vi "Scope_5782_AM_PID.vi"() -> ()   [LabVIEW 2013]
uses:
  <vilib>/userdefined/High Color/nirio_resource_hc.ctl
  FPGA/DataMode.ctl
  <vilib>/Analysis/4window.llb/windowTd.ctl
  Host/Scope/controls/power_spectrum_unit.ctl
  Host/Scope5782/Scope/controls/5782_trigger_type.ctl
  Host/Scope/controls/Data_calc_mode.ctl
  Host/Scope/controls/Data_display_mode.ctl
  Host/Scope/controls/Graph_references.ctl
  Host/Scope/controls/graph_controls.ctl
  Host/Scope/controls/Channel_select.ctl
  Host/Scope5782/Config/FPGAref_5782.ctl
  Host/Communication/response.ctl
  Host/Communication/driver_status.ctl
  Host/Communication/Driver/RemoteConnection/RemoteReferences.ctl
  Host/Communication/Driver/TcpServerDriver/TcpServerDriver.lvclass
  Host/Scope/controls/ScopeMode.ctl
  FPGA/fpga_settings.ctl
  Host/Communication/global_stop.vi
  <vilib>/FPGAPlugInAG/PXIe-7975R/niLvFpga_Open_PXIe-7975R.vi
  <vilib>/rvi/interface/common/dynamic/niFpgaDynamicAddResources.vi
  <vilib>/rvi/interface/common/niFpgaWaitOnOcc.vi
  <vilib>/Utility/error.llb/Error Cluster From Error Code.vi
  <vilib>/rvi/errors/niLvFpgaAdjustHostInterfaceError.vi
  <vilib>/FPGAPlugInAG/Dynamic/niLvFpga_Close_Dynamic.vi
  <vilib>/rvi/interface/nirviOpenFPGA/nirviOpenFPGA.xnode
  FPGA Bitfiles/FPGAmain5782_AM_PID_Tz+TpvSTxoU.lvbitx
  <vilib>/rvi/interface/nirviReadWriteControl/nirviReadWriteControl.xnode
  <vilib>/rvi/FXPMathLib/FxpInterpret/XNode/nifxpmath_Interpret.xnode
  <vilib>/rvi/interface/nirviMethod/nirviMethod.xnode
  <vilib>/rvi/interface/nirviCloseFPGA/nirviCloseFPGA.xnode
  Host/Utilities/Ticker/Ticker.lvclass
  NiFpgaLv.dll
  <vilib>/rvi/interface/Simulation/niFpgaSimulationCallBeginRW.vi
  Host/Communication/Driver/RemoteConnection/RemoteConnection.lvclass
  <vilib>/FPGAPlugInAG/Dynamic/niLvFpga_WriteFifo_Dynamic.vi
  <vilib>/rvi/errors/niLvFpgaMergeErrorWithErrorCode.vi
  <vilib>/Analysis/NI_AALPro.lvlib
panel:
  in  "Ch1 deltaF":bool
  in  "Ch0 deltaF":bool
  in  "Kp":fxp<+/-,32,4>
  in  "Kd/T":fxp<+/-,32,4>
  in  "Ki*T":fxp<+/-,32,4>
  in  "Feedback":bool
  in  "#bins":i32=1 min=1 max=16
  in  "ch1 DC offset":dbl caption="DC offset\nChannel 1"
  in  "ch0 DC offset":dbl caption="DC offset\nChannel 0"
  in  "Output delay delta":dbl(slide) scale=0.0..6.0
  in  "Output delay":dbl(slide) scale=0.0..6.0
  in  "Chart length":i32=200000
  in  "Trigmode":enum32{"Triggered", "Continuous"}(radio)
  in  "Refence for phase":T1
  in  "Graph_refs":T2
  out "Lower chart":dbl[][](graph)
  out "Upper chart":dbl[][](graph)
  out "Lower graph":i16[][](graph)
  in  "Buffer":T4
  in  "Display":T5
  in  "Output mixer fequency [MHz]":dbl
  in  "Trigger":T6
  in  "Ch1 Q":bool
  in  "Ch1 I":bool
  in  "Ch0 Q":bool
  in  "Ch0 I":bool
  in  "Ch1":bool
  in  "Ch0":bool
  out "stop 2":bool
  in  "Zoom freq X":bool
  in  "Zoom freq Y":bool
  in  "Zoom time Y":bool
  in  "Zoom time X":bool
  in  "Unit":T7
  in  "Window":T8=1 items=["Rectangle"=0, "Hanning"=1, "Hamming"=2, "Blackman-Harris"=3, "Exact Blackman"=4, "Blackman"=5, "Flat Top"=6, "4 Term B-Harris "=7, "7 Term B-Harris"=8, "Low Sidelobe"=9, "Blackman Nuttall"=11, "Triangle"=30, "Bartlett-Hanning"=31, "Bohman"=32, "Parzen"=33, "Welch"=34, "Kaiser"=60, "Dolph-Chebyshev"=61, "Gaussian"=62]
  in  "Samples per 5782 record":i32
  in  "Phase offset (deg)":dbl
  in  "Fequency [MHz]":dbl format="%#_8g"
  in  "Mode":T9
  in  "Mixer freq [MHz]":dbl
  out "freqdata":cluster{"f0":dbl, "df":dbl, "magnitude":dbl[]}[](graph)
  out "Upper graph":i16[][](graph)
  in  "Rumode":bool
  in  "Singleshot":bool
  out "error IO":errorcluster
  in  "stop":bool
  in  "resource name":T10="RIO0"
  out "Clocking Option Configured?":bool
  out "Configured?":bool
  # "FPGA setup"
  # "V"
  # "V"
  # "Output delay"
  # "ns"
  # "Auto Zoom"
  # "Output delay delta"
  # "ps"
  # "5782"
  # "Simulated data"
  # "FFT"
  # "Auto Zoom"
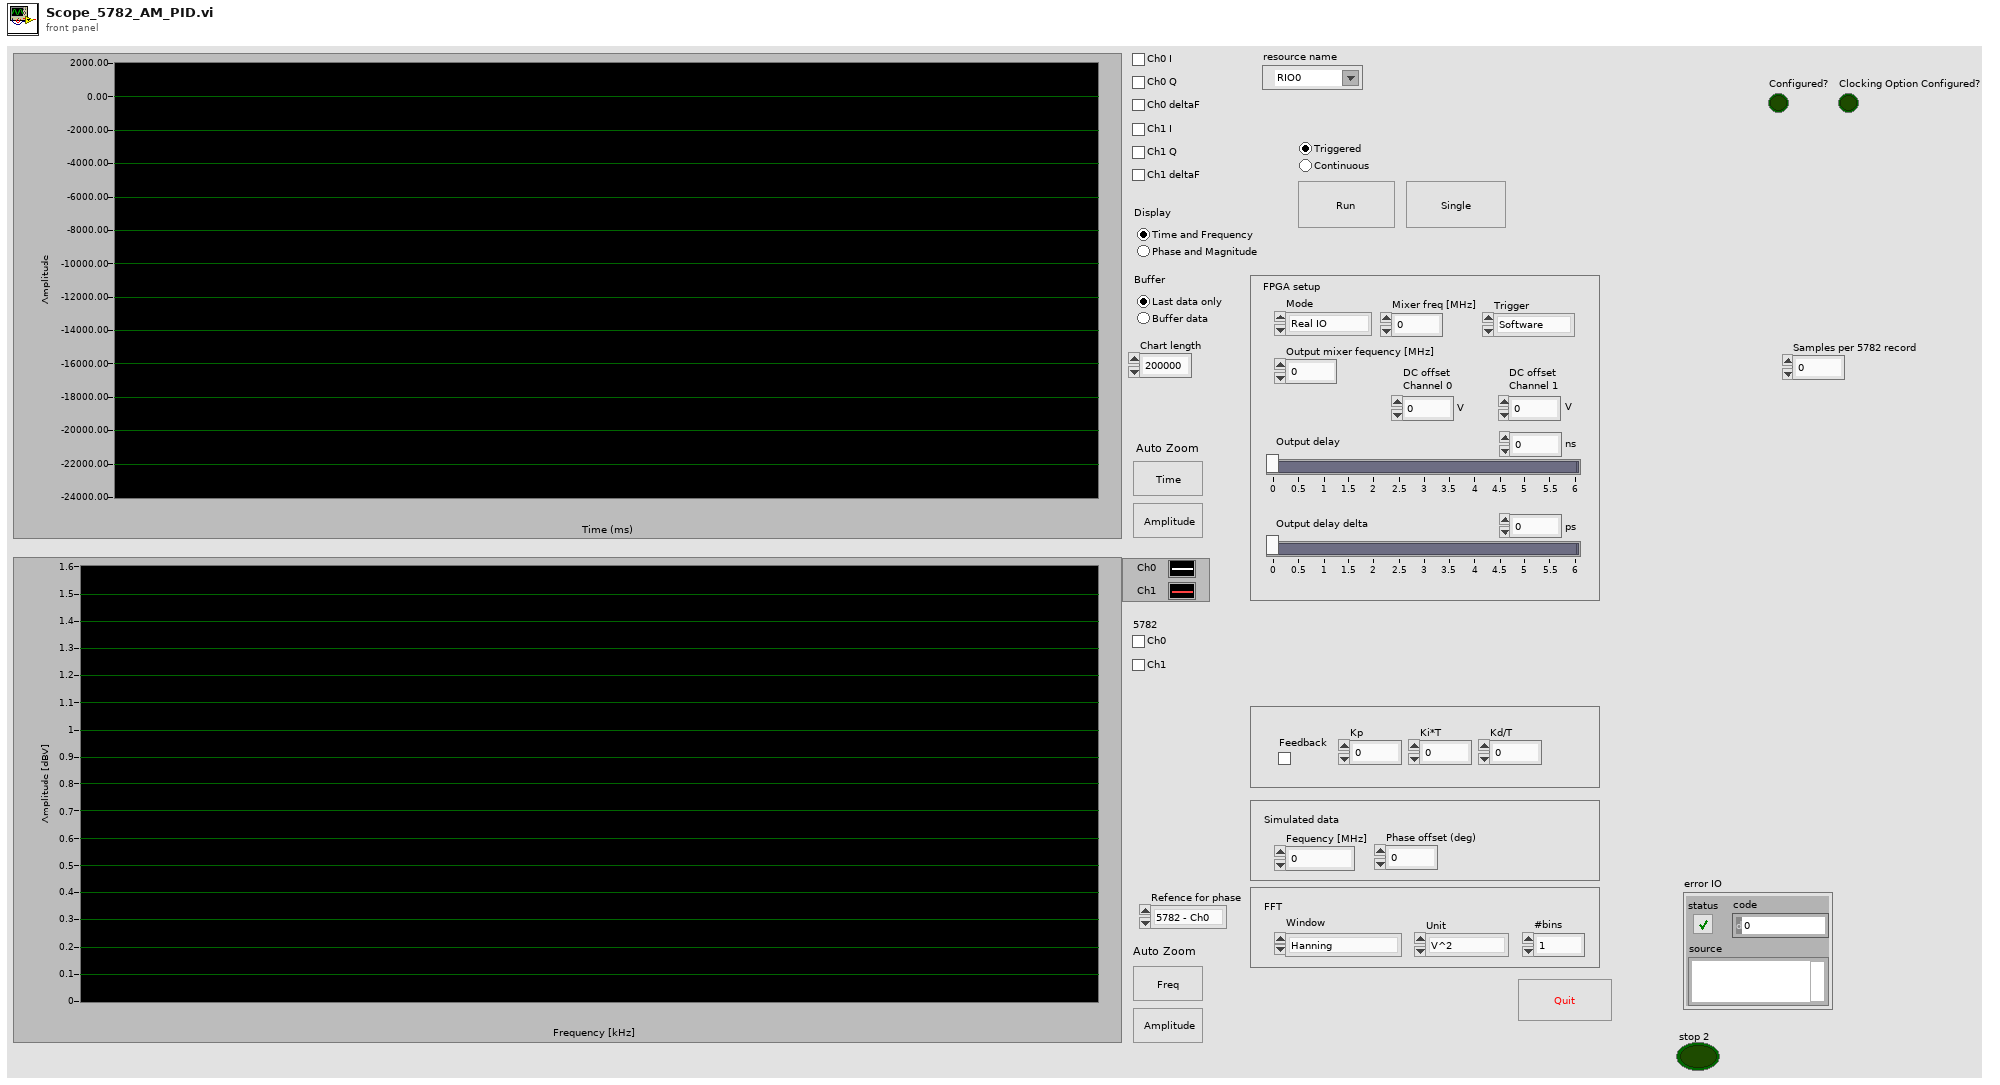
[diagram p1: front panel]
types:
  T1 = typedef "Channel_select.ctl" = enum16{"5782 - Ch0", "5782 - Ch1"}
  T2 = typedef "Graph_references.ctl" = cluster{"upper":T3, "lower":T3, "Freq graph":refnum<vi>}
  T3 = typedef "graph_controls.ctl" = cluster{"Graph":refnum<vi>, "Time btn":refnum<vi>, "Amplitude btn":refnum<vi>, "Chart":refnum<vi>}
  T4 = typedef "Data_display_mode.ctl" = enum32{"Last data only", "Buffer data"}
  T5 = typedef "Data_calc_mode.ctl" = enum32{"Time and Frequency", "Phase and Magnitude"}
  T6 = typedef "5782_trigger_type.ctl" = enum16{"Software", "Trigger input"}
  T7 = typedef "power_spectrum_unit.ctl" = enum16{"V^2", "V", "dBV"}
  T8 = typedef "NI_AALPro.lvlib/windowTd.ctl" = u32
  T9 = typedef "DataMode.ctl" = enum16{"Real IO", "Simulated"}
  T10 = typedef "nirio_resource_hc.ctl" = tag
  T11 = typedef "RemoteConnection.lvclass/RemoteReferences.ctl" = cluster{"a":refnum<vi>, "b":refnum<vi>, "fm":refnum<vi>, "Output delay":refnum<vi>, "Output delay delta":refnum<vi>}
  T12 = typedef "response.ctl" = cluster{"driver status":T13, "Sender":string, "Type":i32, "Variant":variant}
  T13 = typedef "driver_status.ctl" = enum16{"Normal", "Startup", "Connection lost", "Reconnected", "Timeout", "Idle", "Busy"}
  T14 = typedef "FPGAref_5782.ctl" = refnum<k20>
  T15 = enum8{"Internal Clock PLL Off", "Internal Clock PLL On (REF IN)", "External Clock (CLK_IN)", "Internal Clock PLL On (IoModSyncClk)"}
  T16 = typedef "message_queue.ctl" = refnum<queue>
  T17 = typedef "scope_params_5782.ctl" = cluster{"scope mode":T18, "ticker":refnum<class "Ticker.lvclass">, "samples per record":i32, "FPGA ref":T14, "data mode":T9, "5782 Trigger":T6, "Chart length":i32, "RemoteConnection":refnum<class "RemoteConnection.lvclass">, "last phase":dbl[]}
  T18 = typedef "ScopeMode.ctl" = enum16{"Stopped", "Single", "Running", "Continuous"}
  T19 = typedef "fpga_settings.ctl" = enum16{"Feedback Enable", "New FIR coeffs", "FIR shift", "Enable filter", "Set Downsample", "Downsample", "CIC Gain", "Record length", "Trigger samples", "Quiet time", "a_am", "b_am", "Use fixed delay", "fixed sin_fi", "fixed cos_fi", "Ki*Tau", "Kp", "Kd_Tau", "Fi_start", "Fi_delta", "DC_offs 0", "DC_offs 1", "Ki*Tau am", "Kp am", "Kd_Tau am"}
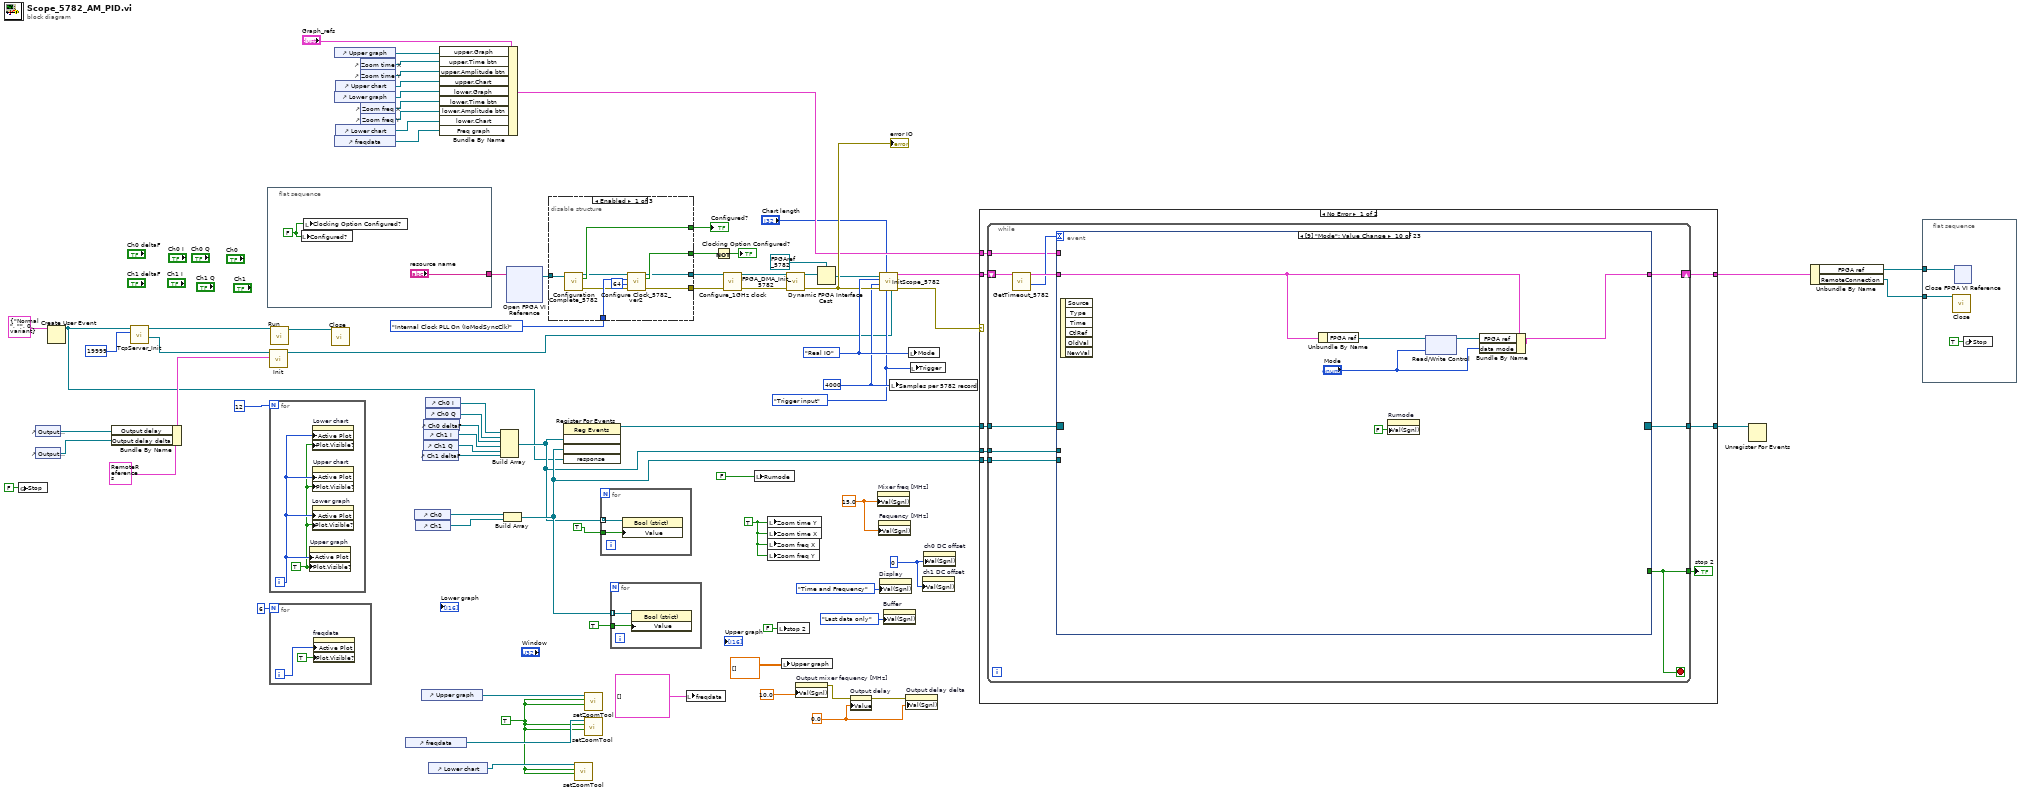
[diagram p0: block diagram]
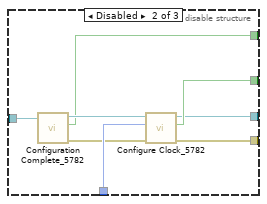
[diagram p2: hidden frame]
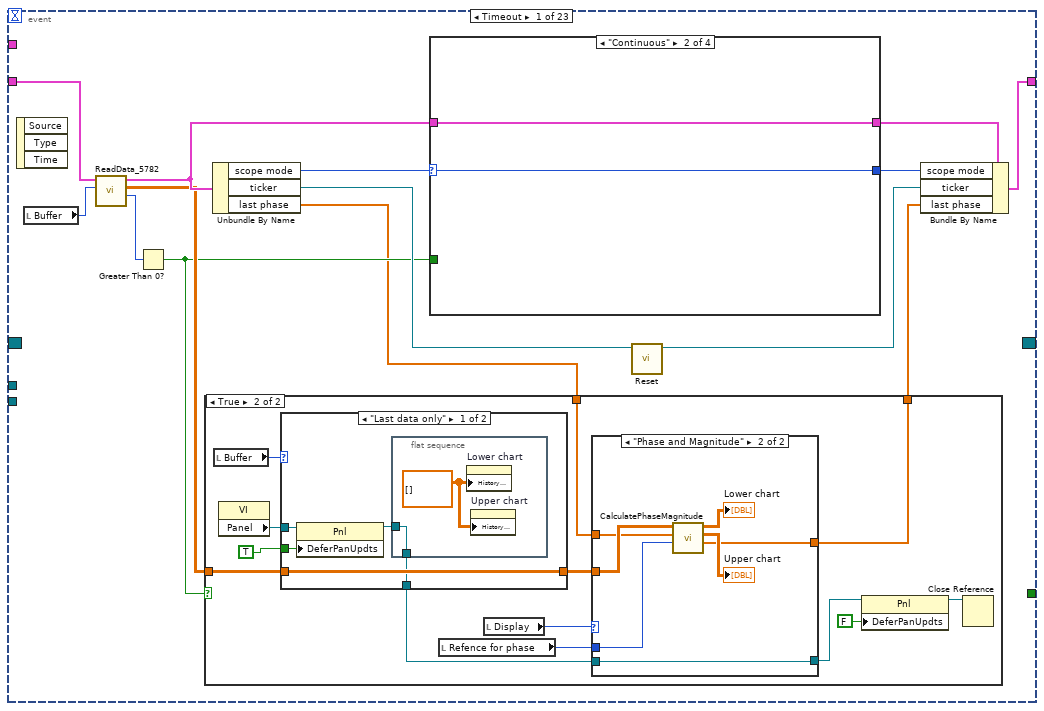
[diagram p4: hidden frame]
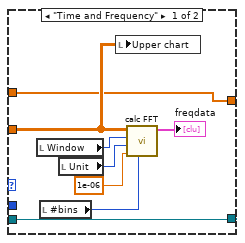
[diagram p7: hidden frame]
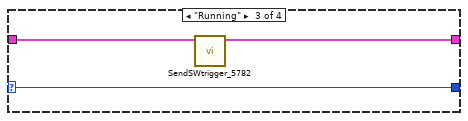
[diagram p9: hidden frame]
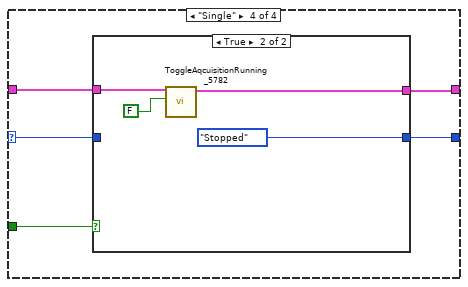
[diagram p10: hidden frame]
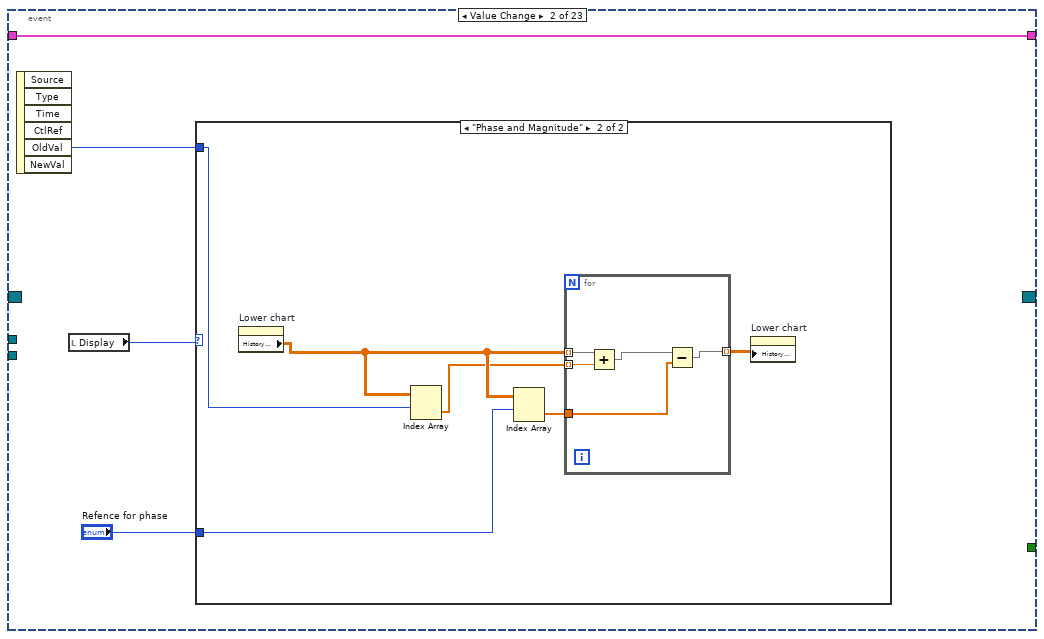
[diagram p12: hidden frame]
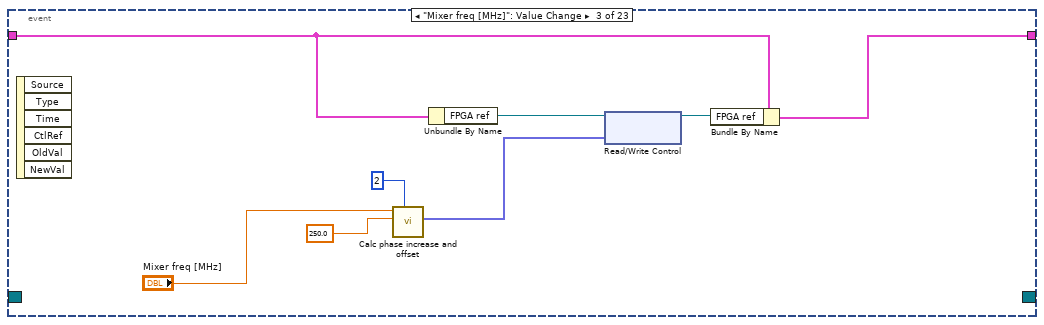
[diagram p14: hidden frame]
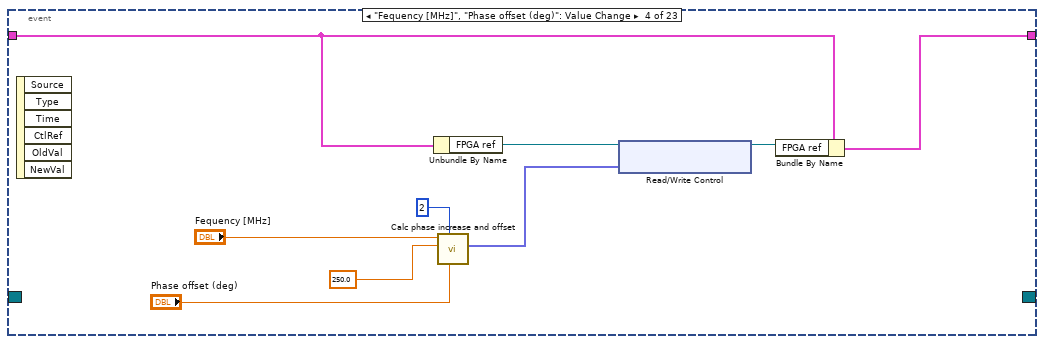
[diagram p15: hidden frame]
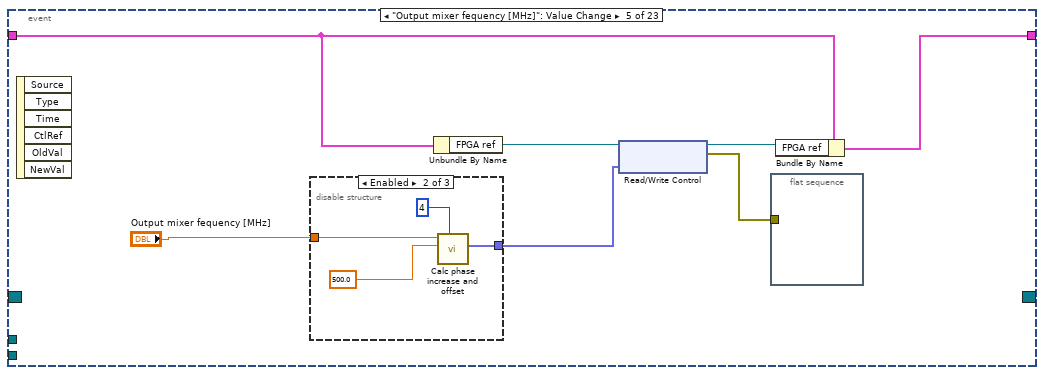
[diagram p16: hidden frame]
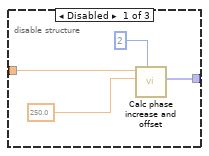
[diagram p17: hidden frame]
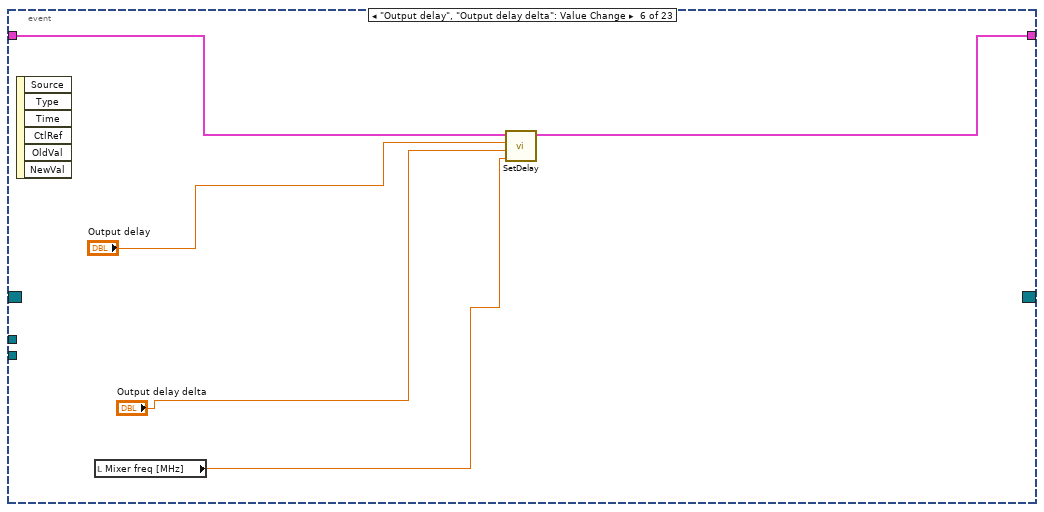
[diagram p19: hidden frame]
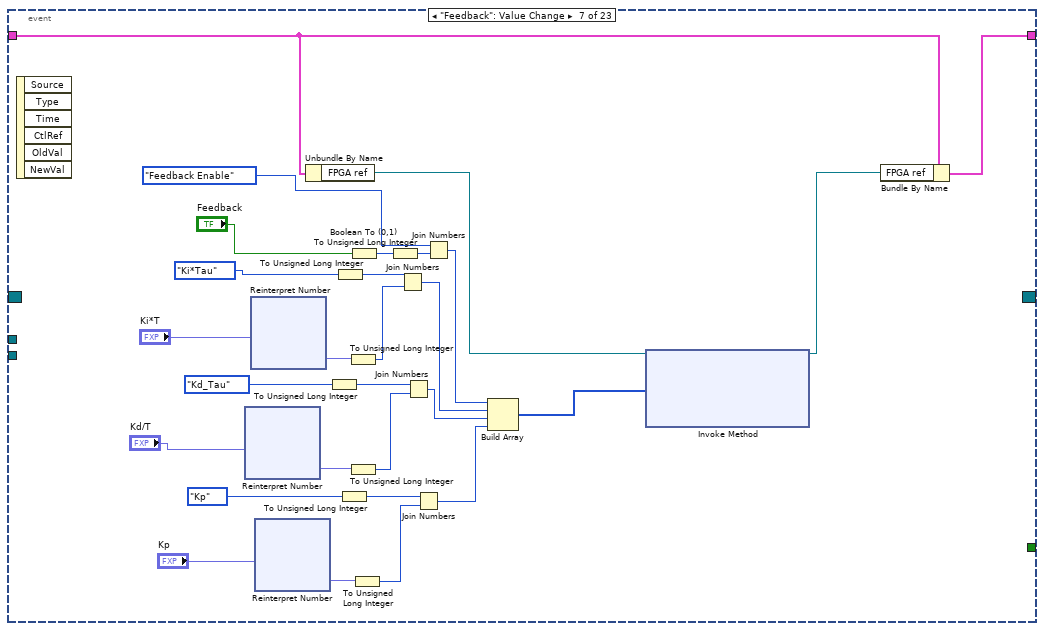
[diagram p20: hidden frame]
diagram:
  w26 = i16 0 ("Value (Signaling)")
  w27 = 0.0 ("Value (Signaling)")
  w49 = 5782_trigger_type."Trigger input" ("Trigger")
  w9 = TRUE ("Zoom  X")
  w64 = TRUE ("Rumode")
  w63 = DataMode."Real IO" ("Mode")
  w51 = 4000 ("Samples to aqcuire")
  w75 = 15.0 ("Mixer requency [MHz]")
  n1 = global write "global_stop.vi" "Stop"(FALSE ("Stop")) -> ()
  n2 = control-ref of="Output delay delta"() -> (w6:refnum<vi>)
  n3 = control-ref of="Output delay"() -> (w5:refnum<vi>)
  n4 = Create User Event(user event datatype=T12 {"driver status"=enum."Normal", "Sender"="", "Type"=0, "Variant"=variant} ("response")) -> (user event=w15:refnum<user-event>)  [unwired: 1 in, 1 out]
  n5 = Bundle By Name(cluster=T11 {"a"=refnum, "b"=refnum, "fm"=refnum, "Output delay"=refnum, "Output delay delta"=refnum} ("refs"), "Output delay"=w6, "Output delay delta"=w5) -> (w22:T11)
  n6 = call "TcpServer_Init.vi"("local port"=u16 19999, "response event"=w15) -> ("Message queue"=w20:T16, "TcpServerDriver"=w17:refnum<class "TcpServerDriver.lvclass">)  [unwired: 8 in]
  n7 = flat-sequence {
    tunnel: ["resource name"] -> w65
    frame #0 {
      w80 = FALSE ("Trigger Acquisition")
      n8 = local write "Configured?"(w80) -> ()
      n9 = local write "Clocking Option Configured?"(w80) -> ()
    }
  }
  n10 = call "Init.vi"("refs"=w22, "server queue"=w20) -> ("RemoteConnection"=w14:refnum<class "RemoteConnection.lvclass">)  [unwired: 9 in]
  n11 = for {
    N: 12 -> [_]
    i -> [w83]
    w82 = TRUE ("Plot.Visible")
    n12 = property on="Upper graph" class="WFGraph (strict)"("Active Plot"=w83, "Plot.Visible?"=w82) -> ()  [unwired: 2 in, 2 out]
    n13 = property on="Lower graph" class="WFGraph (strict)"("Active Plot"=w83, "Plot.Visible?"=w82) -> ()  [unwired: 2 in, 2 out]
    n14 = property on="Lower chart" class="WFChart (strict)"("Active Plot"=w83, "Plot.Visible?"=w82) -> ()  [unwired: 2 in, 2 out]
    n15 = property on="Upper chart" class="WFChart (strict)"("Active Plot"=w83, "Plot.Visible?"=w82) -> ()  [unwired: 2 in, 2 out]
  }
  n16 = for {
    N: 6 -> [_]
    i -> [w84]
    n17 = property on="freqdata" class="WFGraph (strict)"("Active Plot"=w84, "Plot.Visible?"=TRUE ("Plot.Visible")) -> ()  [unwired: 2 in, 2 out]
  }
  n18 = call-dynamic "Run.vi"("BaseDriver in"=w17) -> ("BaseDriver out"=w18:refnum<class "TcpServerDriver.lvclass">)  [unwired: 9 in, 1 out]
  n19 = call-dynamic "Close.vi"("BaseDriver in"=w18) -> ()  [unwired: 9 in, 2 out]
  n20 = control-ref of="Upper graph"() -> (w46:refnum<vi>)
  n21 = control-ref of="Lower graph"() -> (w42:refnum<vi>)
  n22 = control-ref of="freqdata"() -> (w38:refnum<vi>)
  n23 = control-ref of="Upper chart"() -> (w43:refnum<vi>)
  n24 = control-ref of="Lower chart"() -> (w39:refnum<vi>)
  n25 = control-ref of="Zoom time X"() -> (w45:refnum<vi>)
  n26 = control-ref of="Zoom time Y"() -> (w44:refnum<vi>)
  n27 = control-ref of="Zoom freq X"() -> (w41:refnum<vi>)
  n28 = control-ref of="Zoom freq Y"() -> (w40:refnum<vi>)
  n29 = control-ref of="freqdata"() -> (w53:refnum<vi>)
  n30 = control-ref of="Ch0"() -> (w60:refnum<vi>)
  n31 = control-ref of="Ch1"() -> (w61:refnum<vi>)
  n32 = control-ref of="Upper graph"() -> (w54:refnum<vi>)
  n33 = control-ref of="Ch1 deltaF"() -> (w7:refnum<vi>)
  n34 = control-ref of="Ch1 I"() -> (w58:refnum<vi>)
  n35 = control-ref of="Ch1 Q"() -> (w59:refnum<vi>)
  n36 = control-ref of="Ch0 deltaF"() -> (w8:refnum<vi>)
  n37 = control-ref of="Ch0 I"() -> (w56:refnum<vi>)
  n38 = control-ref of="Ch0 Q"() -> (w57:refnum<vi>)
  n39 = control-ref of="Lower chart"() -> (w10:refnum<vi>)
  n40 = Bundle By Name(cluster="Graph_refs", "upper.Graph"=w46, "upper.Time btn"=w45, "upper.Amplitude btn"=w44, "upper.Chart"=w43, "lower.Graph"=w42, "lower.Time btn"=w41, "lower.Amplitude btn"=w40, "lower.Chart"=w39, "Freq graph"=w38) -> (w37:T2)
  n41 = Build Array(w56, w57, w8, w58, w59, w7) -> (w55:refnum<vi>[])
  n42 = Build Array(w60, w61) -> (w67:refnum<vi>[])
  n43 = xnode "Open FPGA VI Reference"("resource name"=w65) -> ("FPGA VI Reference Out"=w32:refnum<k20>)  [unwired: 1 in, 1 out]
  n44 = disable-structure shown="Enabled" {
    disable-tunnel: [w94 w102 _] -> w33
    disable-tunnel: T15."Internal Clock PLL On (IoModSyncClk)" ("Clock Source") -> [w93 w101 _]
    disable-tunnel: [w91 w99 _] -> w3
    disable-tunnel: [w90 w96 w103] -> w4
    disable-tunnel: w32 -> [w86 w98 w103]
    disable-tunnel: [w89 w95 _] -> w30
    frame Enabled {
      n45 = call "Configuration Complete_5782.vi"("FPGA VI Reference in"=w86) -> ("error out"=w92:errorcluster, "Configured?"=w89:bool, "FPGA VI Reference out"=w88:refnum<k20>)  [unwired: 8 in]
      n46 = call "Configure Clock_5782_ver2.vi"("error in"=w92, "User Data 1"=u8 64, "Clock Source"=w93, "FPGA VI Reference"=w88) -> ("error out"=w91:errorcluster, "Configuration Error"=w94:bool, "FPGA VI Reference out"=w90:refnum<k20>)  [unwired: 5 in]
    }
    frame Disabled {
      n47 = call "Configuration Complete_5782.vi"("FPGA VI Reference in"=w98) -> ("error out"=w100:errorcluster, "Configured?"=w95:bool, "FPGA VI Reference out"=w97:refnum<k20>)  [unwired: 8 in]
      n48 = call "Configure Clock_5782.vi"("error in"=w100, "Clock Source"=w101, "FPGA VI Reference in"=w97) -> ("error out"=w99:errorcluster, "Configuration Error"=w102:bool, "FPGA VI Reference Out"=w96:T14)  [unwired: 6 in]
    }
    frame Disabled {
    }
  }
  "Configured?" <- w30
  n49 = register-events(w55, w67, w15) -> (reference out=w71:refnum<event-registration>)  [unwired: 2 in, 1 out]
  n50 = call "setZoomTool.vi"("Zoom Y"=w9, "Zoom  X"=w9, "reference"=w10) -> ()  [unwired: 9 in]
  n51 = call "setZoomTool.vi"("Zoom Y"=w9, "Zoom  X"=w9, "reference"=w53) -> ()  [unwired: 9 in]
  n52 = call "setZoomTool.vi"("Zoom Y"=w9, "Zoom  X"=w9, "reference"=w54) -> ()  [unwired: 9 in]
  n53 = for {
    tunnel: w55 -> [w105] mode=indexing
    tunnel: TRUE ("Rumode") -> [w104]
    n54 = property class="Bool (strict)"(reference=w105, "Value"=w104) -> ()  [unwired: 1 in, 2 out]
  }
  n55 = for {
    tunnel: w67 -> [w107] mode=indexing
    tunnel: TRUE ("Rumode") -> [w106]
    n56 = property class="Bool (strict)"(reference=w107, "Value"=w106) -> ()  [unwired: 1 in, 2 out]
  }
  n57 = local write "freqdata"(cluster{"f0":dbl, "df":dbl, "magnitude":dbl[]}[] [] ("freqdata")) -> ()
  n58 = Not(x=w33) -> (.not. x?=→"Clocking Option Configured?":bool)
  n59 = call "Configure_1GHz clock.vi"("error in"=w3, "FPGA SPI config ref"=w4) -> ("error out"=w2:errorcluster, "FPGA SPI config out"=w1:refnum<k20>)  [unwired: 8 in]
  n60 = local write "Rumode"(FALSE ("Rumode")) -> ()
  n61 = local write "Zoom time Y"(w64) -> ()
  n62 = local write "Zoom time X"(w64) -> ()
  n63 = local write "Zoom freq X"(w64) -> ()
  n64 = local write "Zoom freq Y"(w64) -> ()
  n65 = local write "stop 2"(FALSE ("stop 2")) -> ()
  n66 = local write "Upper graph"(dbl[][] [] ("Timedata")) -> ()
  n67 = call "FPGA_DMA_Init_5782.vi"("error in (no error)"=w2, "FPGA VI Reference"=w1) -> ("error out"=w52:errorcluster, "FPGA VI Out"=w25:refnum<k20>)  [unwired: 7 in, 1 out]
  "error IO" <- w52
  n68 = property on="Output mixer fequency [MHz]" class="DigNum (strict)"("Val(Sgnl)"=10.0 ("Mixer requency [MHz]")) -> (error out=w28:errorcluster)  [unwired: 2 in, 1 out]
  n69 = Dynamic FPGA Interface Cast(Session In=T14 refnum ("FPGA ref"), Type=w25) -> (Session Out=w24:T14)
  n70 = property on="Output delay" class="Slide (strict)"(error in=w28, "Value"=w27) -> (error out=w29:errorcluster)  [unwired: 1 in, 1 out]
  n71 = property on="Mixer freq [MHz]" class="DigNum (strict)"("Val(Sgnl)"=w75) -> ()  [unwired: 2 in, 2 out]
  n72 = property on="Fequency [MHz]" class="DigNum (strict)"("Val(Sgnl)"=w75) -> ()  [unwired: 2 in, 2 out]
  n73 = call "InitScope_5782.vi"("RemoteConnection"=w14, "Trigger"=w49, "Chart length"="Chart length", "error in"=w52, "Samples Per Trigger"=w51, "data mode"=w63, "FPGA ref"=w24) -> ("error out"=w11:errorcluster, "scope params"=w79:T17)  [unwired: 3 in]
  n74 = property on="Display" class="RadioBtnsControl (strict)"("Val(Sgnl)"=Data_calc_mode."Time and Frequency" ("Value (Signaling)")) -> ()  [unwired: 2 in, 2 out]
  n75 = property on="Buffer" class="RadioBtnsControl (strict)"("Val(Sgnl)"=enum32{"Last data only", "Buffer data"}."Last data only" ("Value (Signaling)")) -> ()  [unwired: 2 in, 2 out]
  n76 = local write "Samples per 5782 record"(w51) -> ()
  n77 = property on="Output delay delta" class="Slide (strict)"(error in=w29, "Val(Sgnl)"=w27) -> ()  [unwired: 1 in, 2 out]
  n78 = local write "Mode"(w63) -> ()
  n79 = local write "Trigger"(w49) -> ()
  n80 = property on="ch1 DC offset" class="DigNum (strict)"("Val(Sgnl)"=w26) -> ()  [unwired: 2 in, 2 out]
  n81 = property on="ch0 DC offset" class="DigNum (strict)"("Val(Sgnl)"=w26) -> ()  [unwired: 2 in, 2 out]
  n82 = case shown="No Error" w11 {
    tunnel: w79 -> [w115 w407]
    tunnel: [w114 w407] -> w50
    tunnel: w71 -> [w113 w406]
    tunnel: [w112 w406] -> w70
    tunnel: w55 -> [w111 _]
    tunnel: w67 -> [w110 _]
    tunnel: w37 -> [w108 _]
    frame No Error {
      n83 = while {
        shift-right: [w125] -> w114
        shift-left: w115 -> [w124]
        tunnel: w113 -> [w121]
        tunnel: [w120] -> w112
        tunnel: w111 -> [w119]
        tunnel: w110 -> [w118]
        tunnel: [w117] -> w109
        tunnel: w108 -> [w116]
        stop <- w117 stop-if-true
        n84 = call "GetTimeout_5782.vi"("scope in"=w124) -> ("Time left"=w122:i32, "scope out"=w123:T17)  [unwired: 9 in]
        n85 = event shown="[9] \"Mode\": Value Change" {
          selector: w121 -> [_ _ _ _ _ _ _ _ _ _ _ _ _ _ _ _ _ _ _ _ _ _ _]
          dyn-events: [_ _ _ _ _ _ _ _ _ _ _ _ _ _ _ _ _ _ _ _ _ _ _] -> w120
          timeout: w122 -> [_ _ _ _ _ _ _ _ _ _ _ _ _ _ _ _ _ _ _ _ _ _ _]
          tunnel: [_ _ _ _ _ _ _ _ _ _ _ _ _ _ _ _ _ "stop" _ _ _ _ _] -> w117
          tunnel: w123 -> [w134 w199 w217 w223 w234 w247 w275 w289 w303 w307 w311 w314 w324 w332 w357 w362 w367 w370 w377 w387 w392 w398 w405]
          tunnel: [w137 w199 w215 w222 w233 w246 w274 w288 w302 w306 w310 w313 w321 w329 w357 w362 w366 w370 w377 w387 w392 w398 w405] -> w125
          tunnel: w119 -> [_ _ _ _ _ _ _ _ _ _ _ _ _ _ w356 _ _ _ _ _ _ _ _]
          tunnel: w118 -> [_ _ _ _ _ _ _ _ _ _ _ _ _ _ _ w360 _ _ _ _ _ _ _]
          tunnel: w116 -> [_ _ _ _ _ _ _ _ _ _ _ _ _ _ _ _ _ _ _ _ _ _ w402]
          event Timeout {
            n86 = event-data() -> ()  [unwired: 1 in, 3 out]
            n87 = local read "Buffer"() -> (w128:T4)
            n88 = call "ReadData_5782.vi"("Buffer mode"=w128, "scope params"=w134) -> ("Num elements"=w130:i32, "data"=w131:dbl[][], "scope params out"=w133:T17)  [unwired: 7 in]
            n89 = Greater Than 0?(x=w130) -> (x > 0?=w129:bool)
            n90 = Unbundle By Name(w133) -> ("scope mode"=w136:T18, "ticker"=w139:refnum<class "Ticker.lvclass">, "last phase"=w127:dbl[])
            n91 = case shown="True" w129 {
              tunnel: w131 -> [_ w150]
              tunnel: w127 -> [w140 w142]
              tunnel: [w140 w141] -> w126
              frame False {
              }
              frame True {
                n92 = local read "Buffer"() -> (w152:T4)
                n93 = property class="VI"() -> ("Panel"=w145:refnum<vi>)  [unwired: 2 in, 2 out]
                n94 = case shown="\"Last data only\"" w152 {
                  tunnel: w150 -> [w158 w162]
                  tunnel: [w158 w162] -> w151
                  tunnel: w145 -> [w157 w161]
                  tunnel: TRUE ("Defer Panel Updates") -> [w155 _]
                  tunnel: [w154 w161] -> w143
                  frame "Last data only" {
                    n95 = property class="Pnl"(reference=w157, "DeferPanUpdts"=w155) -> (reference out=w156:refnum<vi>)  [unwired: 1 in, 1 out]
                    n96 = flat-sequence {
                      tunnel: w156 -> [w159]
                      tunnel: [w159] -> w154
                      frame #0 {
                        w160 = dbl[][] [] ("History Data")
                        n97 = property on="Lower chart" class="WFChart (strict)"("History Data"=w160) -> ()  [unwired: 2 in, 2 out]
                        n98 = property on="Upper chart" class="WFChart (strict)"("History Data"=w160) -> ()  [unwired: 2 in, 2 out]
                      }
                    }
                  }
                  frame "Buffer data" {
                  }
                }
                n99 = local read "Refence for phase"() -> (w149:T1)
                n100 = local read "Display"() -> (w153:T5)
                n101 = case shown="\"Phase and Magnitude\"" w153 {
                  tunnel: w151 -> [w166 w177]
                  tunnel: w149 -> [_ w174]
                  tunnel: [w165 w173] -> w147
                  tunnel: w143 -> [w165 w173]
                  tunnel: w142 -> [w163 w172]
                  tunnel: [w163 w171] -> w141
                  frame "Time and Frequency" {
                    n102 = local read "Window"() -> (w167:T8)
                    n103 = local read "#bins"() -> (w164:i32)
                    n104 = local read "Unit"() -> (w168:T7)
                    n105 = local write "Upper chart"(w166) -> ()
                    n106 = call "calc FFT.vi"("#bins"=w164, "dt"=1e-06, "Unit"=w168, "Window"=w167, "data"=w166) -> ("Power Spectrum / PSD"=→"freqdata":cluster{"f0":dbl, "df":dbl, "magnitude":dbl[]}[])  [unwired: 6 in]
                  }
                  frame "Phase and Magnitude" {
                    n107 = call "CalculatePhaseMagnitude.vi"("phase reference channel"=w174, "previous phase"=w172, "data"=w177) -> ("last phase"=w171:dbl[], "Magnitude"=→"Upper chart":dbl[][], "Phase"=→"Lower chart":dbl[][])  [unwired: 6 in]
                  }
                }
                n108 = property class="Pnl"(reference=w147, "DeferPanUpdts"=FALSE ("Defer Panel Updates")) -> (reference out=w146:refnum<vi>)  [unwired: 1 in, 1 out]
                n109 = Close Reference(reference=w146) -> ()  [unwired: 1 in, 1 out]
              }
            }
            n110 = case shown="\"Continuous\"" w136 {
              selector: w136 -> [w179 w181 w184 w185]
              tunnel: [w179 w181 w184 w189] -> w135
              tunnel: w133 -> [w178 w180 w183 w187]
              tunnel: [w178 w180 w182 w186] -> w132
              tunnel: w129 -> [_ _ _ w188]
              frame "Stopped" {
              }
              frame "Continuous" {
              }
              frame "Running" {
                n111 = call "SendSWtrigger_5782.vi"("scope in"=w183) -> ("scope out"=w182:T17)  [unwired: 9 in, 1 out]
              }
              frame "Single" {
                n112 = case shown="True" w188 {
                  tunnel: [w190 ScopeMode."Stopped" ("scope mode")] -> w189
                  tunnel: w187 -> [w191 w194]
                  tunnel: [w191 w193] -> w186
                  tunnel: w185 -> [w190 _]
                  frame False {
                  }
                  frame True {
                    n113 = call "ToggleAqcuisitionRunning_5782.vi"("Acquisition running"=FALSE, "scope in"=w194) -> ("scope out"=w193:T17)  [unwired: 8 in, 1 out]
                  }
                }
              }
            }
            n114 = call "Reset.vi"("Ticker in"=w139) -> ("Ticker out"=w138:refnum<class "Ticker.lvclass">)  [unwired: 9 in, 1 out]
            n115 = Bundle By Name(cluster=w132, "scope mode"=w135, "ticker"=w138, "last phase"=w126) -> (w137:T17)
          }
          event Value Change {
            n116 = event-data() -> ("OldVal"=w196:T1)  [unwired: 1 in, 5 out]
            n117 = local read "Display"() -> (w197:T5)
            n118 = case shown="\"Phase and Magnitude\"" w197 {
              tunnel: "Refence for phase" -> [_ w204]
              tunnel: w196 -> [_ w202]
              frame "Time and Frequency", Default {
              }
              frame "Phase and Magnitude" {
                n119 = property on="Lower chart" class="WFChart (strict)"() -> ("History Data"=w203:dbl[][])  [unwired: 2 in, 2 out]
                n120 = Index Array(array=w203, index (row)=w202) -> (element=w201:dbl[])  [unwired: 1 in]
                n121 = Index Array(array=w203, index (row)=w204) -> (element=w205:dbl[])  [unwired: 1 in]
                n122 = for {
                  tunnel: w203 -> [w208] mode=indexing
                  tunnel: w205 -> [w210]
                  tunnel: [w209] -> w200 mode=indexing
                  tunnel: w201 -> [w207] mode=indexing
                  n123 = Add(x=w208, y=w207) -> (x+y=w206:dbl[])
                  n124 = Subtract(x=w206, y=w210) -> (x-y=w209:dbl[])
                }
                n125 = property on="Lower chart" class="WFChart (strict)"("History Data"=w200) -> ()  [unwired: 2 in, 2 out]
              }
            }
          }
          event "Mixer freq [MHz]": Value Change {
            n126 = event-data() -> ()  [unwired: 1 in, 6 out]
            n127 = call "Calc phase increase and offset.vi"("# of DDS"=2, "fclk (MHz)"=250.0 ("fclk (800MHz)"), "f_generated (MHz)"="Mixer freq [MHz]") -> ("Phase out"=w211:fxp<+,64,64>[])  [unwired: 6 in, 2 out]
            n128 = Unbundle By Name(w217) -> ("FPGA ref"=w218:T14)
            n129 = xnode "Read/Write Control"("FPGA VI Reference In"=w218, "Phase 5782"=w211) -> ("FPGA VI Reference Out"=w216:T14)  [unwired: 1 in, 1 out]
            n130 = Bundle By Name(cluster=w217, "FPGA ref"=w216) -> (w215:T17)
          }
          event "Fequency [MHz]", "Phase offset (deg)": Value Change {
            n131 = event-data() -> ()  [unwired: 1 in, 6 out]
            n132 = Unbundle By Name(w223) -> ("FPGA ref"=w225:T14)
            n133 = call "Calc phase increase and offset.vi"("Phase offset (deg)"="Phase offset (deg)", "# of DDS"=2, "fclk (MHz)"=250.0 ("fclk (800MHz)"), "f_generated (MHz)"="Fequency [MHz]") -> ("Phase out"=w219:fxp<+,64,64>[])  [unwired: 5 in, 2 out]
            n134 = xnode "Read/Write Control"("FPGA VI Reference In"=w225, "Simulated phase 5782"=w219) -> ("FPGA VI Reference Out"=w224:T14)  [unwired: 1 in, 1 out]
            n135 = Bundle By Name(cluster=w223, "FPGA ref"=w224) -> (w222:T17)
          }
          event "Output mixer fequency [MHz]": Value Change {
            n136 = event-data() -> ()  [unwired: 1 in, 6 out]
            n137 = disable-structure shown="Enabled" {
              disable-tunnel: [w236 w240 _] -> w230
              disable-tunnel: "Output mixer fequency [MHz]" -> [w235 w239 _]
              frame Disabled {
                n138 = call "Calc phase increase and offset.vi"("# of DDS"=2, "fclk (MHz)"=250.0 ("fclk (800MHz)"), "f_generated (MHz)"=w235) -> ("Phase out"=w236:fxp<+,64,64>[])  [unwired: 6 in, 2 out]
              }
              frame Enabled {
                n139 = call "Calc phase increase and offset.vi"("# of DDS"=4, "fclk (MHz)"=500.0 ("fclk (800MHz)"), "f_generated (MHz)"=w239) -> ("Phase out"=w240:fxp<+,64,64>[])  [unwired: 6 in, 2 out]
              }
              frame Disabled {
              }
            }
            n140 = Unbundle By Name(w234) -> ("FPGA ref"=w229:T14)
            n141 = xnode "Read/Write Control"("FPGA VI Reference In"=w229, "Phase output"=w230) -> ("FPGA VI Reference Out"=w228:T14, "error out"=w231:errorcluster)  [unwired: 1 in]
            n142 = flat-sequence {
              tunnel: w231 -> [_]
              frame #0 {
              }
            }
            n143 = Bundle By Name(cluster=w234, "FPGA ref"=w228) -> (w233:T17)
          }
          event "Output delay", "Output delay delta": Value Change {
            n144 = event-data() -> ()  [unwired: 1 in, 6 out]
            n145 = local read "Mixer freq [MHz]"() -> (w243:dbl)
            n146 = call "SetDelay.vi"("Mixer freq [MHz]"=w243, "Output delay delta"="Output delay delta", "Output delay"="Output delay", "scope in"=w247) -> ("scope out"=w246:T17)  [unwired: 7 in]
          }
          event "Feedback": Value Change {
            n147 = event-data() -> ()  [unwired: 1 in, 6 out]
            n148 = xnode "Reinterpret Number"("x"="Kd/T") -> ("y"=w261:fxp<+,32,32>)
            n149 = xnode "Reinterpret Number"("x"="Ki*T") -> ("y"=w258:fxp<+,32,32>)
            n150 = xnode "Reinterpret Number"("x"="Kp") -> ("y"=w265:fxp<+,32,32>)
            n151 = Unbundle By Name(w275) -> ("FPGA ref"=w273:T14)
            n152 = To Unsigned Long Integer(number=fpga_settings."Kd_Tau" ("FPGA Setting")) -> (unsigned 32bit integer=w259:u32)
            n153 = To Unsigned Long Integer(number=fpga_settings."Ki*Tau" ("FPGA Setting")) -> (unsigned 32bit integer=w255:u32)
            n154 = To Unsigned Long Integer(number=fpga_settings."Kp" ("FPGA Setting")) -> (unsigned 32bit integer=w262:u32)
            n155 = To Unsigned Long Integer(number=w258) -> (unsigned 32bit integer=w254:u32)
            n156 = To Unsigned Long Integer(number=w261) -> (unsigned 32bit integer=w260:u32)
            n157 = Boolean To (0,1)(Boolean="Feedback") -> (0, 1=w270:i16)
            n158 = To Unsigned Long Integer(number=w265) -> (unsigned 32bit integer=w264:u32)
            n159 = To Unsigned Long Integer(number=w270) -> (unsigned 32bit integer=w267:u32)
            n160 = Join Numbers(hi=w255, lo=w254) -> ((hi.lo)=w253:u64)
            n161 = Join Numbers(hi=w259, lo=w260) -> ((hi.lo)=w252:u64)
            n162 = Join Numbers(hi=w262, lo=w264) -> ((hi.lo)=w272:u64)
            n163 = Join Numbers(hi=fpga_settings."Feedback Enable" ("FPGA Setting"), lo=w267) -> ((hi.lo)=w268:u64)
            n164 = Build Array(w268, w253, w252, w272) -> (w271:u64[])
            n165 = xnode "Invoke Method"("FPGA VI Reference In"=w273, "Data"=w271) -> ("FPGA VI Reference Out"=w248:T14)  [unwired: 2 in, 2 out]
            n166 = Bundle By Name(cluster=w275, "FPGA ref"=w248) -> (w274:T17)
          }
          event "ch0 DC offset": Value Change {
            n167 = event-data() -> ()  [unwired: 1 in, 6 out]
            n168 = Unbundle By Name(w289) -> ("FPGA ref"=w277:T14)
            n169 = Divide(x=32768, y=5) -> (x/y=w286:dbl)
            n170 = Multiply(x="ch0 DC offset", y=w286) -> (x*y=w285:dbl)
            n171 = Round To Nearest(number=w285) -> (nearest integer value=w284:dbl)
            n172 = To Word Integer(number=w284) -> (16bit integer=w278:i16)
            n173 = xnode "Reinterpret Number"("x"=w278) -> ("y"=w281:fxp<+/-,16,14>)
            n174 = xnode "Reinterpret Number"("x"=w281) -> ("y"=w280:fxp<+,16,16>)
            n175 = call "Write 16bit value.vi"("value"=w280, "FPGA Setting"=fpga_settings."DC_offs 0", "FPGA ref"=w277) -> ("FPGA ref out"=w276:T14)  [unwired: 7 in, 1 out]
            n176 = Bundle By Name(cluster=w289, "FPGA ref"=w276) -> (w288:T17)
          }
          event "ch1 DC offset": Value Change {
            n177 = event-data() -> ()  [unwired: 1 in, 6 out]
            n178 = Unbundle By Name(w303) -> ("FPGA ref"=w291:T14)
            n179 = Divide(x=32768, y=5) -> (x/y=w300:dbl)
            n180 = Multiply(x="ch1 DC offset", y=w300) -> (x*y=w299:dbl)
            n181 = Round To Nearest(number=w299) -> (nearest integer value=w298:dbl)
            n182 = To Word Integer(number=w298) -> (16bit integer=w292:i16)
            n183 = xnode "Reinterpret Number"("x"=w292) -> ("y"=w295:fxp<+/-,16,14>)
            n184 = xnode "Reinterpret Number"("x"=w295) -> ("y"=w294:fxp<+,16,16>)
            n185 = call "Write 16bit value.vi"("value"=w294, "FPGA Setting"=fpga_settings."DC_offs 1", "FPGA ref"=w291) -> ("FPGA ref out"=w290:T14)  [unwired: 7 in, 1 out]
            n186 = Bundle By Name(cluster=w303, "FPGA ref"=w290) -> (w302:T17)
          }
          event Value Change {
            n187 = event-data() -> ()  [unwired: 1 in, 6 out]
            n188 = Unbundle By Name(w307) -> ("FPGA ref"=w309:T14)
            n189 = property on="Rumode" class="Bool (strict)"("Val(Sgnl)"=FALSE ("Value (Signaling)")) -> ()  [unwired: 2 in, 2 out]
            n190 = xnode "Read/Write Control"("FPGA VI Reference In"=w309, "Mode"="Mode") -> ("FPGA VI Reference Out"=w308:T14)  [unwired: 1 in, 1 out]
            n191 = Bundle By Name(cluster=w307, "FPGA ref"=w308, "data mode"="Mode") -> (w306:T17)
          }
          event Value Change {
            n192 = event-data() -> ()  [unwired: 1 in, 6 out]
            n193 = Bundle By Name(cluster=w311, "5782 Trigger"="Trigger") -> (w310:T17)
          }
          event "Samples per 5782 record": Value Change {
            n194 = event-data() -> ()  [unwired: 1 in, 6 out]
            n195 = Unbundle By Name(w314) -> ("FPGA ref"=w317:T14)
            n196 = xnode "Read/Write Control"("FPGA VI Reference In"=w317, "5782 record length"="Samples per 5782 record") -> ("FPGA VI Reference Out"=w316:T14)  [unwired: 1 in, 1 out]
            n197 = Bundle By Name(cluster=w314, "FPGA ref"=w316, "samples per record"="Samples per 5782 record") -> (w313:T17)
          }
          event "Singleshot": Value Change {
            n198 = event-data() -> ()  [unwired: 1 in, 6 out]
            n199 = local write "Rumode"(FALSE ("Rumode")) -> ()
            n200 = Bundle By Name(cluster=w324, "scope mode"=ScopeMode."Single") -> (w319:T17)
            n201 = call "ToggleContinousMode.vi"("Cont Acquisition"=FALSE, "scope in"=w319) -> ("scope out"=w318:T17)  [unwired: 8 in, 1 out]
            n202 = call "ToggleAqcuisitionRunning_5782.vi"("Acquisition running"=TRUE, "scope in"=w318) -> ("scope out"=w322:T17)  [unwired: 8 in, 1 out]
            n203 = call "SendSWtrigger_5782.vi"("scope in"=w322) -> ("scope out"=w321:T17)  [unwired: 9 in, 1 out]
          }
          event "Rumode": Value Change {
            n204 = event-data() -> ()  [unwired: 1 in, 6 out]
            n205 = case shown="\"Triggered\"" "Trigmode" {
              tunnel: [ScopeMode."Running" ("scope mode") ScopeMode."Continuous" ("scope mode")] -> w327
              frame "Triggered" {
              }
              frame "Continuous" {
              }
            }
            n206 = Select(t=w327, s="Rumode", f=ScopeMode."Stopped" ("scope mode")) -> (s? t:f=w331:T18)
            n207 = Bundle By Name(cluster=w332, "scope mode"=w331) -> (w330:T17)
            n208 = case shown="\"Single\", \"Running\"" w331 {
              tunnel: w330 -> [w339 w346 w350]
              tunnel: [w340 w344 w351] -> w329
              frame "Single", "Running" {
                n209 = call "ToggleContinousMode.vi"("Cont Acquisition"=FALSE, "scope in"=w339) -> ("scope out"=w337:T17)  [unwired: 8 in, 1 out]
                n210 = call "ToggleAqcuisitionRunning_5782.vi"("Acquisition running"=TRUE, "scope in"=w337) -> ("scope out"=w341:T17)  [unwired: 8 in, 1 out]
                n211 = call "SendSWtrigger_5782.vi"("scope in"=w341) -> ("scope out"=w340:T17)  [unwired: 9 in, 1 out]
              }
              frame "Continuous" {
                n212 = call "ToggleAqcuisitionRunning_5782.vi"("Acquisition running"=TRUE, "scope in"=w346) -> ("scope out"=w345:T17)  [unwired: 8 in, 1 out]
                n213 = call "ToggleContinousMode.vi"("Cont Acquisition"=TRUE ("Acquisition running"), "scope in"=w345) -> ("scope out"=w344:T17)  [unwired: 8 in, 1 out]
              }
              frame "Stopped" {
                n214 = call "ToggleContinousMode.vi"("Cont Acquisition"=FALSE, "scope in"=w350) -> ("scope out"=w348:T17)  [unwired: 8 in, 1 out]
                n215 = call "ToggleAqcuisitionRunning_5782.vi"("Acquisition running"=FALSE, "scope in"=w348) -> ("scope out"=w351:T17)  [unwired: 8 in, 1 out]
              }
            }
          }
          event Value Change {
            n216 = event-data() -> ("CtlRef"=w355:refnum<vi>, "NewVal"=w353:bool)  [unwired: 1 in, 4 out]
            n217 = Search 1D Array(1D array=w356, element=w355) -> (index of element=w354:i32)  [unwired: 1 in]
            n218 = property on="Upper graph" class="WFGraph (strict)"("Active Plot"=w354, "Plot.Visible?"=w353) -> ()  [unwired: 2 in, 2 out]
            n219 = property on="Upper chart" class="WFChart (strict)"("Active Plot"=w354, "Plot.Visible?"=w353) -> ()  [unwired: 2 in, 2 out]
          }
          event Value Change {
            n220 = event-data() -> ("CtlRef"=w361:refnum<vi>, "NewVal"=w358:bool)  [unwired: 1 in, 4 out]
            n221 = Search 1D Array(1D array=w360, element=w361) -> (index of element=w359:i32)  [unwired: 1 in]
            n222 = property on="freqdata" class="WFGraph (strict)"("Active Plot"=w359, "Plot.Visible?"=w358) -> ()  [unwired: 2 in, 2 out]
            n223 = property on="Lower chart" class="WFChart (strict)"("Active Plot"=w359, "Plot.Visible?"=w358) -> ()  [unwired: 2 in, 2 out]
          }
          event User Event {
            n224 = event-data() -> ("Sender"=w365:string, "Variant"=w364:variant, "driver status"=w363:T13)  [unwired: 1 in, 5 out]
            n225 = Unbundle By Name(w367) -> ("RemoteConnection"=w369:refnum<class "RemoteConnection.lvclass">)
            n226 = call "HandleRemoteMessage.vi"("driver status"=w363, "Message data"=w364, "Sender"=w365, "RemoteConnection in"=w369) -> ("RemoteConnection out"=w368:refnum<class "RemoteConnection.lvclass">)  [unwired: 6 in, 1 out]
            n227 = Bundle By Name(cluster=w367, "RemoteConnection"=w368) -> (w366:T17)
          }
          event "stop": Value Change {
            n228 = event-data() -> ()  [unwired: 1 in, 6 out]
          }
          event Value Change {
            n229 = event-data() -> ()  [unwired: 1 in, 6 out]
            n230 = case shown="\"V\"" "Unit" {
              tunnel: ["V" "dBV" "V^2"] -> w374
              frame "V" {
              }
              frame "dBV" {
              }
              frame "V^2" {
              }
            }
            n231 = Concatenate Strings("Amplitude [", w374, "]") -> (w372:string)
            n232 = property on="freqdata" class="WFGraph (strict)"("YScale.NameLbl.Text"=w372) -> ()  [unwired: 2 in, 2 out]
          }
          event "#bins": Value Change {
            n233 = event-data() -> ()  [unwired: 1 in, 6 out]
            n234 = local read "Upper chart"() -> (w383:dbl[][])
            n235 = local read "Window"() -> (w384:T8)
            n236 = local read "Unit"() -> (w385:T7)
            n237 = call "calc FFT.vi"("#bins"="#bins", "dt"=1e-06, "Unit"=w385, "Window"=w384, "data"=w383) -> ("Power Spectrum / PSD"=w382:cluster{"f0":dbl, "df":dbl, "magnitude":dbl[]}[])  [unwired: 6 in]
            n238 = local write "freqdata"(w382) -> ()
          }
          event "Zoom time X", "Zoom time Y": Value Change {
            n239 = event-data() -> ()  [unwired: 1 in, 6 out]
            n240 = control-ref of="Upper chart"() -> (w390:refnum<vi>)
            n241 = control-ref of="Upper graph"() -> (w391:refnum<vi>)
            n242 = call "setZoomTool.vi"("Zoom Y"="Zoom time Y", "Zoom  X"="Zoom time X", "reference"=w390) -> ()  [unwired: 9 in]
            n243 = call "setZoomTool.vi"("Zoom Y"="Zoom time Y", "Zoom  X"="Zoom time X", "reference"=w391) -> ()  [unwired: 9 in]
          }
          event "Zoom freq Y", "Zoom freq X": Value Change {
            n244 = event-data() -> ()  [unwired: 1 in, 6 out]
            n245 = control-ref of="Lower chart"() -> (w396:refnum<vi>)
            n246 = control-ref of="Lower graph"() -> (w395:refnum<vi>)
            n247 = control-ref of="freqdata"() -> (w397:refnum<vi>)
            n248 = call "setZoomTool.vi"("Zoom Y"="Zoom freq Y", "Zoom  X"="Zoom freq X", "reference"=w397) -> ()  [unwired: 9 in]
            n249 = call "setZoomTool.vi"("Zoom Y"="Zoom freq Y", "Zoom  X"="Zoom freq X", "reference"=w396) -> ()  [unwired: 9 in]
            n250 = call "setZoomTool.vi"("Zoom Y"="Zoom freq Y", "Zoom  X"="Zoom freq X", "reference"=w395) -> ()  [unwired: 9 in]
          }
          event Value Change {
            w401 = dbl[][] [] ("History Data")
            n251 = event-data() -> ()  [unwired: 1 in, 6 out]
            n252 = property on="Upper chart" class="WFChart (strict)"("History Data"=w401) -> ()  [unwired: 2 in, 2 out]
            n253 = property on="Lower chart" class="WFChart (strict)"("History Data"=w401) -> ()  [unwired: 2 in, 2 out]
            n254 = local write "freqdata"(cluster{"f0":dbl, "df":dbl, "magnitude":dbl[]}[] [] ("freqdata")) -> ()
            n255 = call "UpdateGraphs.vi"("Buffer mode"="Buffer", "Display mode"="Display", "Graph_refs"=w402) -> ()  [unwired: 9 in]
            n256 = property on="Zoom time X" class="Bool (strict)"("Val(Sgnl)"=TRUE ("Value (Signaling)")) -> ()  [unwired: 2 in, 2 out]
          }
        }
      }
      "stop 2" <- w109
    }
    frame Error {
    }
  }
  n257 = Unregister For Events(event registration refnum=w70) -> ()  [unwired: 1 in, 1 out]
  n258 = Unbundle By Name(w50) -> ("FPGA ref"=w78:T14, "RemoteConnection"=w13:refnum<class "RemoteConnection.lvclass">)
  n259 = flat-sequence {
    tunnel: w78 -> [w410]
    tunnel: w13 -> [w409]
    frame #0 {
      n260 = call "Close.vi"("RemoteConnection in"=w409) -> ()  [unwired: 9 in, 2 out]
      n261 = xnode "Close FPGA VI Reference"("FPGA VI Reference In"=w410) -> ()  [unwired: 1 in, 1 out]
      n262 = global write "global_stop.vi" "Stop"(TRUE ("Stop")) -> ()
    }
  }
